vi "Wait.vi"(3 "error in (no error)":errorcluster, 4 "wait, ms":u32) -> (9 "error out":errorcluster)   [LabVIEW 2017]
doc: "This SubVI perform ms delay with predefined period"
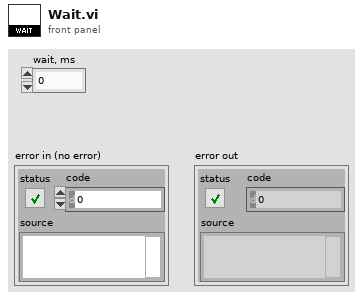
[diagram p1: front panel]
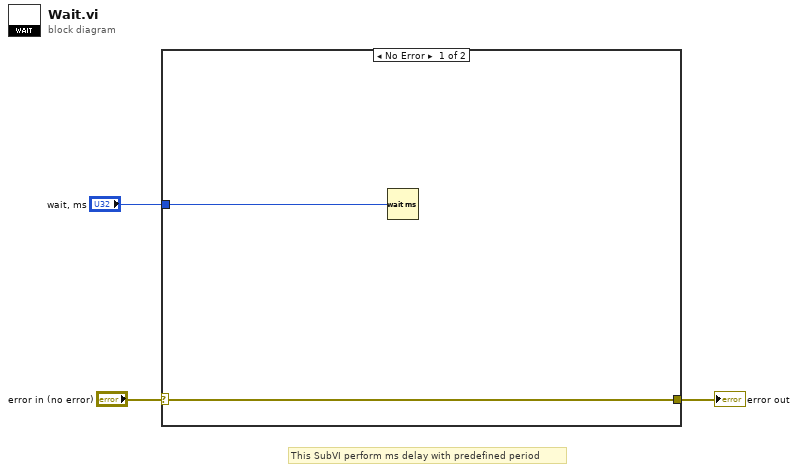
[diagram p0: block diagram]
diagram:
  # "This SubVI perform ms delay with predefined period"
  n1 = case shown="No Error" "error in (no error)" {
    selector: "error in (no error)" -> [w5 w6]
    tunnel: [w5 w6] -> w2
    tunnel: "wait, ms" -> [w4 _]
    frame No Error {
      n2 = Wait (ms)(milliseconds to wait=w4) -> ()  [unwired: 1 out]
    }
    frame Error {
    }
  }
  "error out" <- w2
